vi "sounds.vi"() -> ()   [LabVIEW 2012]
uses:
  <vilib>/sound2/lvsound2.llb/Sound Data Format.ctl
  <vilib>/sound2/lvsound2.llb/Sampling Mode.ctl
  <vilib>/Platform/TimedLoop/XDataNode/timing_clust.ctl
  <vilib>/Platform/TimedLoop/XDataNode/nitl_modes.ctl
  <vilib>/Platform/TimedLoop/XDataNode/wakeup.ctl
  <vilib>/sound2/lvsound2.llb/Sound Output Set Volume (Single).vi
  <vilib>/sound2/lvsound2.llb/Sound Output Write (DBL Single).vi
  <vilib>/Platform/TimedLoop/XDataNode/XDataNode.xnode
  <vilib>/Platform/TimedLoop/XDataNode/XDNodeRunTimeDep.lvlib
panel:
  out "Waveform Graph":waveform(dbl)(graph)
  in  "Sound Format":T1={"sample rate (S/s)"=44100.0, "number of channels"=2, "bits per sample"=16}
  in  "Device ID":u32
  in  "Volume":dbl(slide)=70.40816326530613 scale=0.0..100.0
  in  "Test":bool
  in  "stop":bool
  # "Sounds VI"
  # "This VI is used to generate a \"ding\" sound on command from trialrunner.vi running on the realtime target.   This VI is run on the windows host, which has access to sound, and communicates with the real-time via network shared variables."
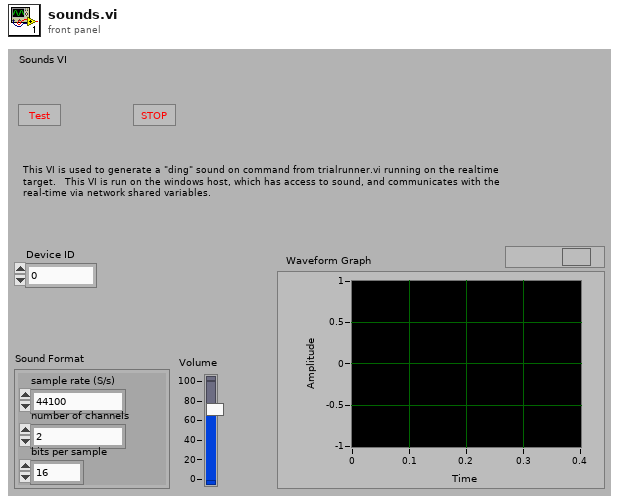
[diagram p1: front panel]
types:
  T1 = typedef "Sound Data Format.ctl" = cluster{"sample rate (S/s)":dbl, "number of channels":i32, "bits per sample":i32}
  T2 = typedef "Sampling Mode.ctl" = i32
  T3 = typedef "Sound Output Task ID.ctl" = u32
  T4 = typedef "XDNodeRunTimeDep.lvlib/timing_clust.ctl" = cluster{"Expected End [f-1]":u64, "Actual End [f-1]":u64, "Finished Late? [f-1]":bool, "Expected End [i-1]":u64, "Actual End [i-1]":u64, "Finished Late? [i-1]":bool, "Expected Start [i]":u64, "Actual Start [i]":u64, "Expected Start [f]":u64, "Actual Start [f]":u64, "Source Name":string, "Structure Name":string, "Period":i64, "Deadline":i64, "Offset":i64, "Start":i64, "Priority":i32, "Timeout":i32, "Mode":T5, "Wakeup Reason":T6, "Error":errorcluster, "Source Type":string, "Secondary Source Type":string, "Global End Time":u64, "Global Start Time":u64, "Frame Duration":u64, "Iteration Duration":u64, "Assigned CPU":i32, "I/O Scan Engine Mode":u32}
  T5 = typedef "XDNodeRunTimeDep.lvlib/nitl_modes.ctl" = enum32{"No Change", "Process missed periods, maintain original phase", "Discard missed periods, maintain original phase", "Process missed periods, ignore original phase", "Discard missed periods, ignore original phase"}
  T6 = typedef "XDNodeRunTimeDep.lvlib/wakeup.ctl" = enum32{"Normal", "Aborted", "Asynchronous wakeup", "Timing source error", "Timed loop error", "Timeout"}
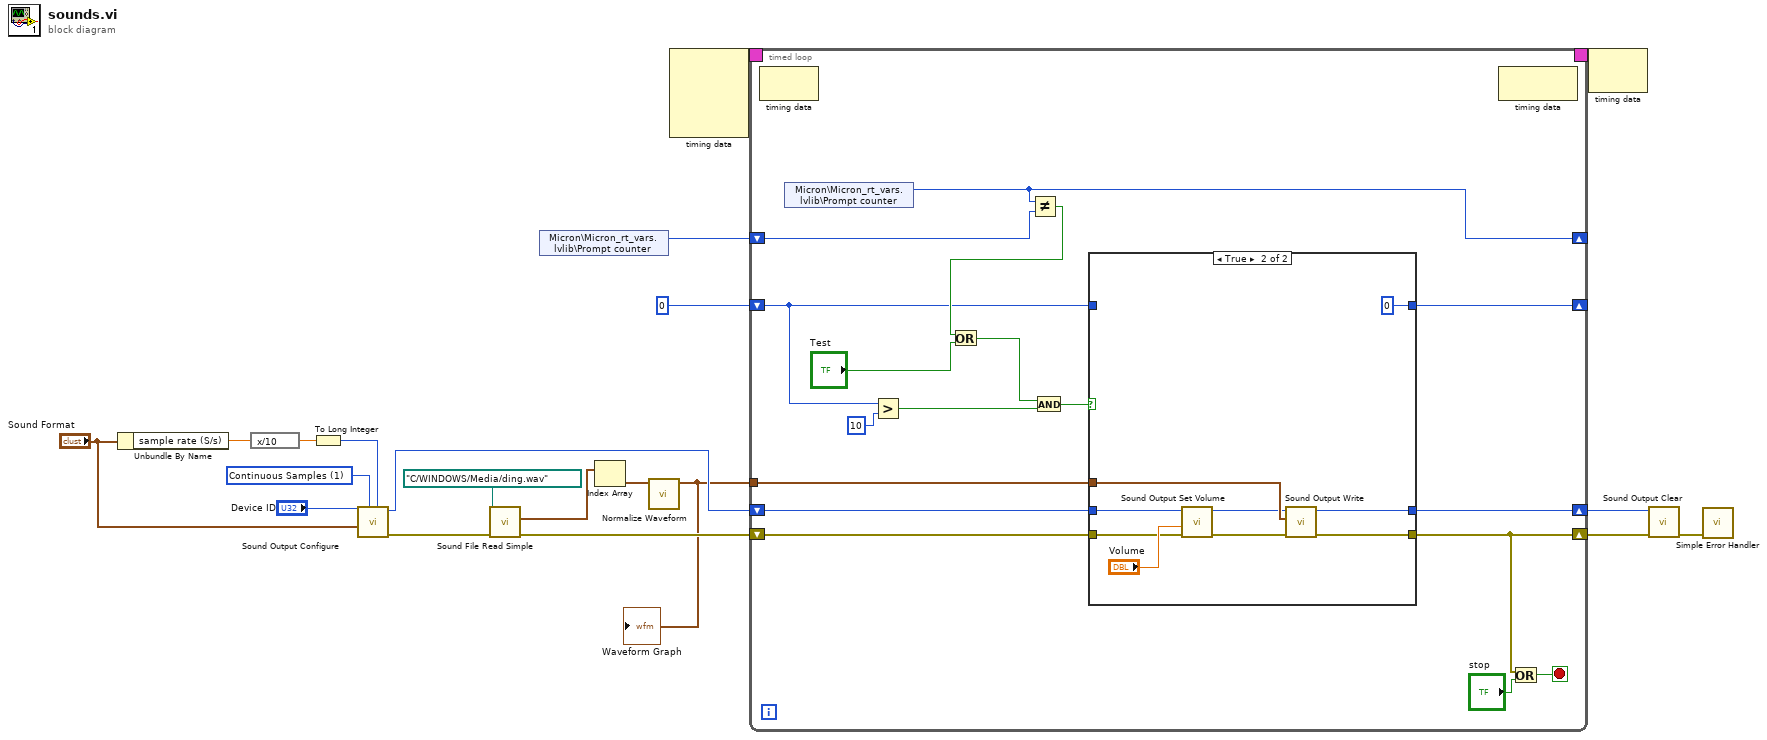
[diagram p0: block diagram]
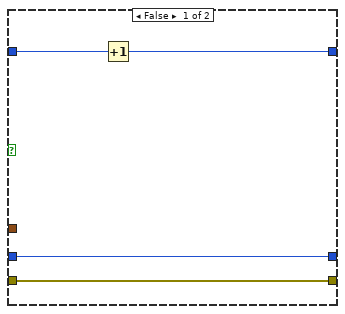
[diagram p2: hidden frame]
diagram:
  w9 = T2 1 items=["Finite Samples", "Continuous Samples"] ("sample mode")
  n1 = Unbundle By Name("Sound Format") -> ("sample rate (S/s)"=w11:dbl)
  n2 = expression code="x/10"(w11) -> (w13:dbl)
  n3 = To Long Integer(number=w13) -> (32bit integer=w12:i32)
  n4 = call <vilib>:"Sound Output Configure.vi"("number of samples/ch"=w12, "sample mode"=w9, "sound format"="Sound Format", "device ID"="Device ID") -> ("error out"=w5:errorcluster, "task ID"=w10:T3)  [unwired: 2 in, 4 out]
  n5 = call <vilib>:"Sound File Read Simple.vi"("error in (no error)"=w5, "path"=path "C:/WINDOWS/Media/ding.wav") -> ("error out"=w4:errorcluster, "data"=w3:waveform(dbl)[])  [unwired: 6 in, 2 out]
  n6 = shared-variable "Micron\\Micron_rt_vars.lvlib\\Prompt counter"() -> (w17:u32)  [unwired: 2 out]
  n7 = Index Array(array=w3) -> (element=w2:waveform(dbl))  [unwired: 1 in]
  n8 = call <vilib>:"Normalize Waveform.vi"("waveform in"=w2) -> ("normalized waveform"=w1:waveform(dbl))  [unwired: 7 in, 3 out]
  "Waveform Graph" <- w1
  n9 = node-c288() -> (w20:T4)  [unwired: 4 out]
  n10 = timed-loop {
    timing: w20 -> [_]
    timing-out: [_] -> w19
    shift-right: [w29] -> _
    shift-left: 0 -> [w28]
    shift-right: [w30] -> _
    shift-left: w17 -> [w32]
    shift-right: [w23] -> w8
    shift-left: w10 -> [w21]
    shift-right: [w25] -> w7
    shift-left: w4 -> [w22]
    tunnel: w1 -> [w24]
    stop <- w26 stop-if-true
    n11 = node-c288() -> ()  [unwired: 2 out]
    n12 = shared-variable "Micron\\Micron_rt_vars.lvlib\\Prompt counter"() -> (w30:u32)  [unwired: 2 out]
    n13 = Greater?(x=w28, y=10) -> (0:w36:bool)
    n14 = Not Equal?(x=w30, y=w32) -> (x != y?=w31:bool)
    n15 = Or(x=w31, y="Test") -> (x .or. y?=w34:bool)
    n16 = And(x=w34, y=w36) -> (x .and. y?=w35:bool)
    n17 = case shown="True" w35 {
      tunnel: [w40 0] -> w29
      tunnel: w28 -> [w41 _]
      tunnel: [w39 w49] -> w25
      tunnel: w22 -> [w39 w45]
      tunnel: w24 -> [_ w48]
      tunnel: w21 -> [w38 w44]
      tunnel: [w38 w47] -> w23
      frame False {
        n18 = Increment(x=w41) -> (x+1=w40:i32)
      }
      frame True {
        n19 = call-poly <vilib>:"Sound Output Set Volume.vi"("error in (no error)"=w45, "volume"="Volume", "task ID"=w44) -> ("error out"=w43:errorcluster, "task ID out"=w42:T3)  [unwired: 7 out]
        n20 = call-poly <vilib>:"Sound Output Write.vi"("error in (no error)"=w43, "data"=w48, "task ID"=w42) -> ("error out"=w49:errorcluster, "task ID out"=w47:T3)  [unwired: 1 in, 6 out]
      }
    }
    n21 = node-c288() -> ()  [unwired: 2 out]
    n22 = Or(x=w25, y="stop") -> (x .or. y?=w26:bool)
  }
  n23 = node-c288(w19) -> ()  [unwired: 1 out]
  n24 = call <vilib>:"Sound Output Clear.vi"("error in (no error)"=w7, "task ID"=w8) -> ("error out"=w15:errorcluster)  [unwired: 9 out]
  n25 = call <vilib>:"Simple Error Handler.vi"("error in (no error)"=w15) -> ()  [unwired: 1 in, 8 out]
